vi "Vector - Complex.vi"(7 "data type of variable":cdb[](array[numeric]), 8 "error in":errorcluster, 10 "variable name":string, 11 "pipe in":T1) -> (0 "error out":errorcluster, 2 "value":cdb[](array[numeric]) format="%.2f", 3 "pipe out":T1)   [LabVIEW 2013, in "GOLPI library.lvlib"]
uses:
  GOLPI library.lvlib
  LV Process.lvlibp/Pipe Handle.ctl
  <vilib>/Utility/error.llb/Error Cluster From Error Code.vi
  <vilib>/ErrorRing/Error Ring.xnode
  LV Process.lvlibp
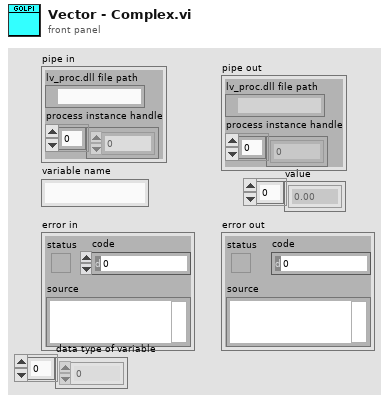
[diagram p1: front panel]
types:
  T1 = typedef "LV Process.lvlibp/Pipe Handle.ctl" = cluster{"lv_proc.dll file path":path, "process instance handle":u32[]}
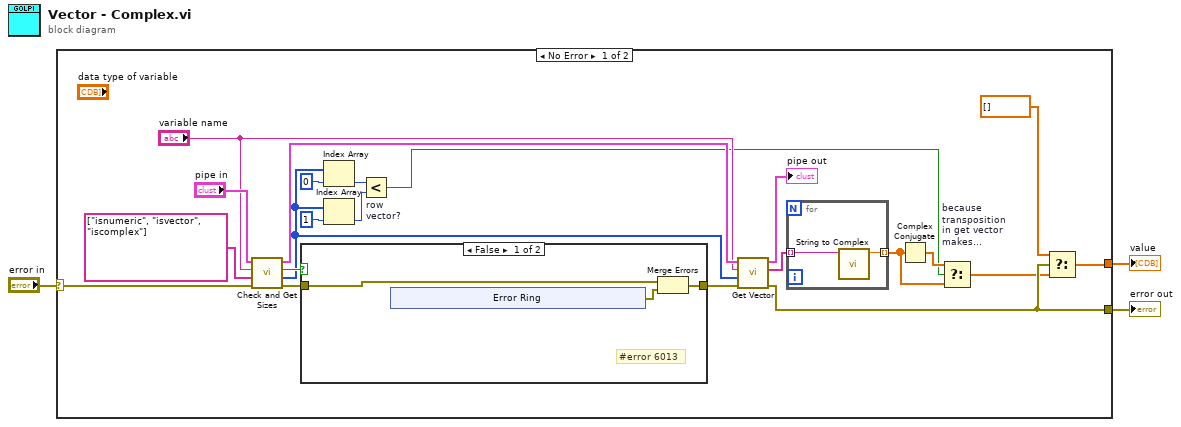
[diagram p0: block diagram]
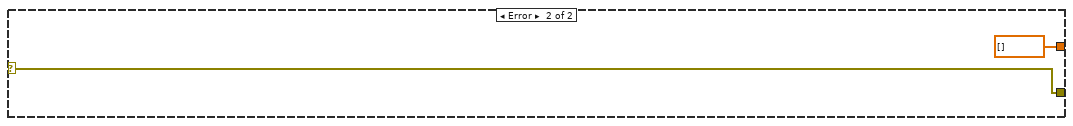
[diagram p3: hidden frame]
diagram:
  n1 = case shown="No Error" "error in" {
    selector: "error in" -> [w21 w38]
    tunnel: [w14 w38] -> w3
    tunnel: [w24 cdb[] [] ("value")] -> w1
    frame No Error {
      n2 = call "Check and Get Sizes.vi"("error in (no error)"=w21, "test commands"=string[] ["isnumeric", "isvector", "iscomplex"], "variable name"="variable name", "pipe in"="pipe in") -> ("error out"=w20:errorcluster, "octave sizes"=w8:i32[], "all tests OK?"=w22:bool, "pipe out"=w18:T1)  [unwired: 4 in]
      n3 = case shown="False" w22 {
        tunnel: w20 -> [w29 w36]
        tunnel: [w28 w36] -> w15
        frame False {
          # "#error 6013"
          n4 = xnode "Error Ring"() -> ("error out"=w30:errorcluster)
          n5 = Merge Errors(w29, w30) -> (w28:errorcluster)
        }
        frame True {
        }
      }
      n6 = Index Array(array=w8, index=0) -> (element=w10:i32)
      n7 = Index Array(array=w8, index=1) -> (element=w9:i32)
      n8 = Less? "row\nvector?"(x=w10, y=w9) -> (x < y?=w4:bool)
      n9 = call "Get Vector.vi"("error in (no error)"=w15, "octave vector sizes"=w8, "variable name"="variable name", "pipe in"=w18) -> ("error out"=w14:errorcluster, "vector"=w13:string[], "pipe out"=→"pipe out":T1)  [unwired: 5 in]
      n10 = for {
        tunnel: w13 -> [w27] mode=indexing
        tunnel: [w26] -> w6 mode=indexing
        n11 = call "String to Complex.vi"("string"=w27) -> ("complex number"=w26:cdb)  [unwired: 10 in]
      }
      n12 = Complex Conjugate(1:w6) -> (0:w7:cdb[])
      n13 = Select "because\ntransposition\nin get vector\nmakes\nconjugate"(t=w7, s=w4, f=w6) -> (s? t:f=w5:cdb[])
      n14 = Select(t=cdb[] [] ("value"), s=w14, f=w5) -> (s? t:f=w24:cdb[])
    }
    frame Error {
    }
  }
  "value" <- w1
  "error out" <- w3
